vi "Pan speed (SubVI).vi"(9 "valid":bool, 11 "pan in":dbl format="%#_13g") -> (1 "millisecond timer value":u32, 2 "degree/sec":dbl, 3 "speed":dbl)   [LabVIEW 2016]
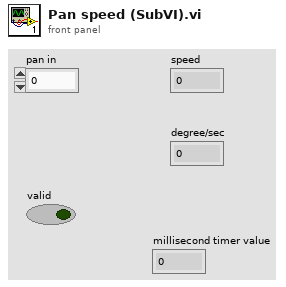
[diagram p1: front panel]
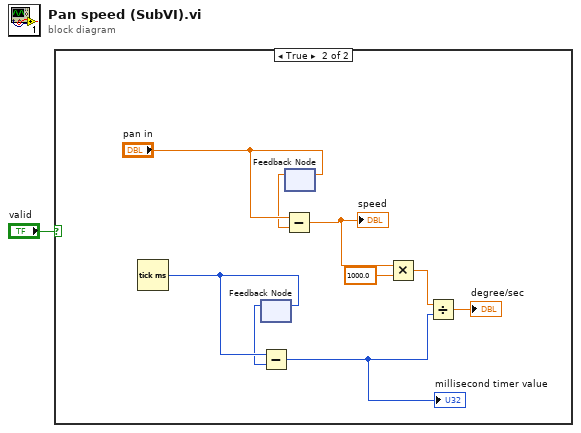
[diagram p0: block diagram]
diagram:
  n1 = case shown="True" "valid" {
    frame False {
    }
    frame True {
      n2 = Tick Count (ms)() -> (millisecond timer value=w8:u32)
      n3 = feedback #1() -> (w7:u32)  [unwired: 1 in]
      n4 = feedback-in #1(w8) -> ()
      n5 = Subtract(x=w8, y=w7) -> (x-y=w2:u32)
      "millisecond timer value" <- w2
      n6 = feedback #2() -> (w9:dbl)  [unwired: 1 in]
      n7 = Subtract(x="pan in", y=w9) -> (x-y=w6:dbl)
      "speed" <- w6
      n8 = feedback-in #2("pan in") -> ()
      n9 = Multiply(x=w6, y=1000.0) -> (x*y=w4:dbl)
      n10 = Divide(x=w4, y=w2) -> (x/y=→"degree/sec":dbl)
    }
  }
